vi "ConvertSpeedRefernce.vi"(9 "channels":T2[](array[typedef]), 10 "node properties":T1[](array[typedef]), 11 "dg properties in":T1[](array[typedef])) -> (3 "dg properties out":T1[](array[typedef]))   [LabVIEW 2017, in "ServerComm.lvlib"]
uses:
  <vilib>/addons/InsightCM/Devices/Shared/Common/ServerComm/ServerComm.lvlib
  <vilib>/addons/InsightCM/MessageBus/Base/controls/R2_Channel.ctl
  <vilib>/addons/InsightCM/MessageBus/Base/controls/KeyValuePair.ctl
  <vilib>/addons/InsightCM/MessageBus/Base/controls/Metric.ctl
  <vilib>/addons/InsightCM/Utilities/PropertyHelpers/PropertyHelpers.lvlib
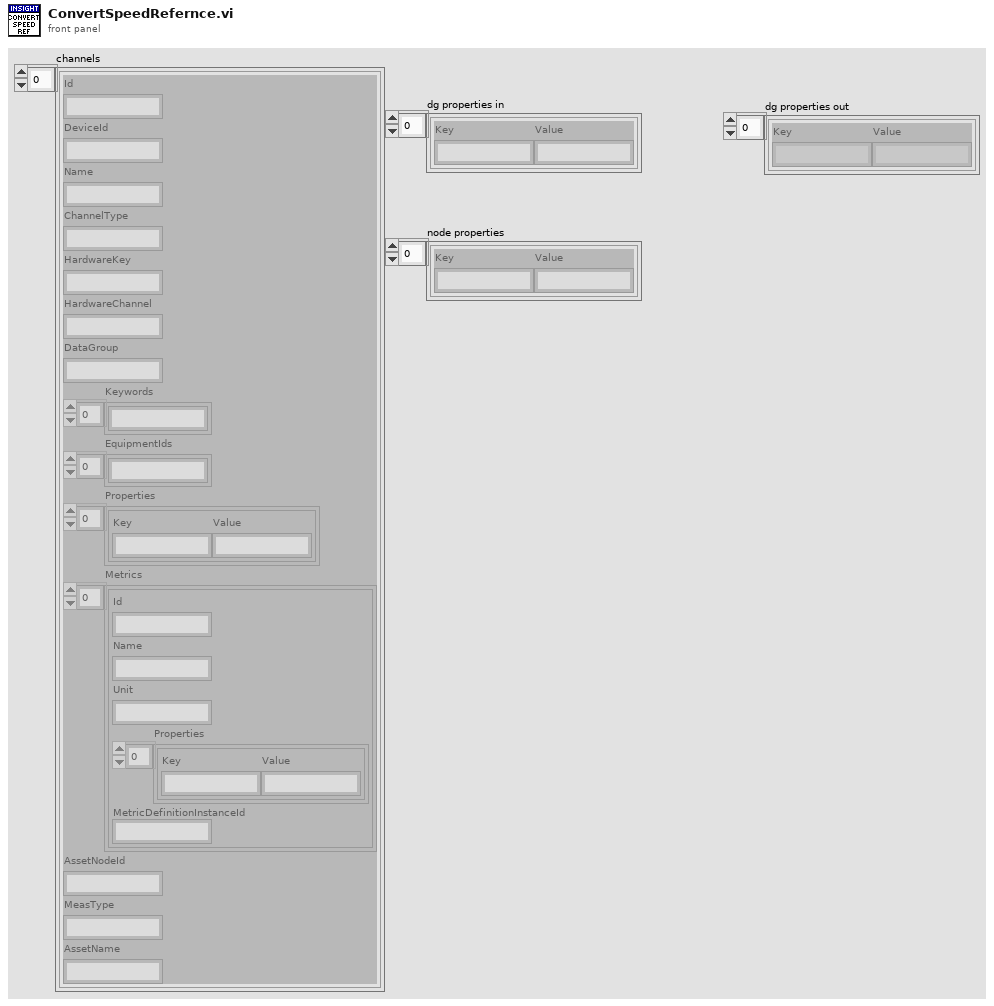
[diagram p1: front panel]
types:
  T1 = typedef "KeyValuePair.ctl" = cluster{"Key":string, "Value":string}
  T2 = typedef "R2_Channel.ctl" = cluster{"Id":string, "DeviceId":string, "Name":string, "ChannelType":string, "HardwareKey":string, "HardwareChannel":string, "DataGroup":string, "Keywords":string[], "EquipmentIds":string[], "Properties":T1[], "Metrics":T3[], "AssetNodeId":string, "MeasType":string, "AssetName":string}
  T3 = typedef "Metric.ctl" = cluster{"Id":string, "Name":string, "Unit":string, "Properties":T1[], "MetricDefinitionInstanceId":string}
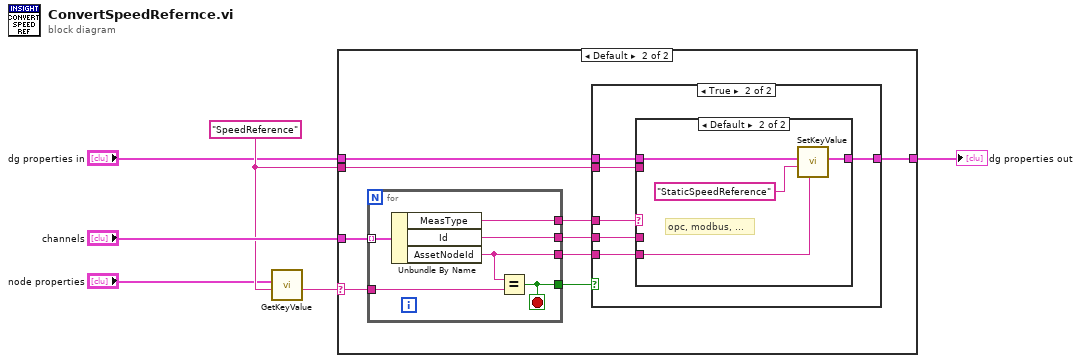
[diagram p0: block diagram]
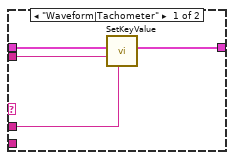
[diagram p4: hidden frame]
diagram:
  w4 = "SpeedReference" ("key")
  n1 = call <vilib>:"GetKeyValue.vi"("key"=w4, "key value pairs"="node properties") -> ("value"=w5:string)  [unwired: 7 in, 2 out]
  n2 = case shown="Default" w5 {
    selector: w5 -> [_ w15]
    tunnel: "channels" -> [_ w16]
    tunnel: "dg properties in" -> [w7 w13]
    tunnel: w4 -> [_ w12]
    tunnel: [w7 w10] -> w1
    frame "" {
    }
    frame Default {
      n3 = for {
        tunnel: w16 -> [w37] mode=indexing
        tunnel: w15 -> [w36]
        tunnel: [w35] -> w14
        tunnel: [w34] -> w11
        tunnel: [w33] -> w9
        tunnel: [w32] -> w8
        stop <- w35 stop-if-true
        n4 = Unbundle By Name(w37) -> ("MeasType"=w33:string, "Id"=w34:string, "AssetNodeId"=w32:string)
        n5 = Equal?(x=w32, y=w36) -> (x = y?=w35:bool)
      }
      n6 = case shown="True" w14 {
        tunnel: w13 -> [w17 w23]
        tunnel: w12 -> [_ w22]
        tunnel: w11 -> [_ w21]
        tunnel: [w17 w20] -> w10
        tunnel: w9 -> [_ w19]
        tunnel: w8 -> [_ w18]
        frame False {
        }
        frame True {
          n7 = case shown="Default" w19 {
            tunnel: w23 -> [w27 w31]
            tunnel: w22 -> [w26 _]
            tunnel: w21 -> [w25 _]
            tunnel: [w24 w30] -> w20
            tunnel: w18 -> [_ w28]
            frame "Waveform|Tachometer" {
              n8 = call <vilib>:"SetKeyValue.vi"("value"=w25, "key"=w26, "key value pairs"=w27) -> ("key value pairs out"=w24:T1[])  [unwired: 8 in]
            }
            frame Default {
              # "opc, modbus, ..."
              n9 = call <vilib>:"SetKeyValue.vi"("value"=w28, "key"="StaticSpeedReference", "key value pairs"=w31) -> ("key value pairs out"=w30:T1[])  [unwired: 8 in]
            }
          }
        }
      }
    }
  }
  "dg properties out" <- w1
